vi "Get-Ctrl-Ref's & Label's.vi"(0 "VI Refnum":refnum<vi>, 7 "Show All Label List":bool, 11 "error in (no error)":errorcluster) -> (4 "Quick-GUI-Update out":refnum<class "Quick-GUI-Update.lvclass">, 8 "Label's List":string[][](array[string]), 15 "error out":errorcluster)   [LabVIEW 2020, in "Easy GUI Operation.lvlib" / "Quick-GUI-Update.lvclass"]
uses:
  Quick-GUI-Update.lvclass
  Quick-GUI-Update.lvclass/Quick-GUI-Update.ctl
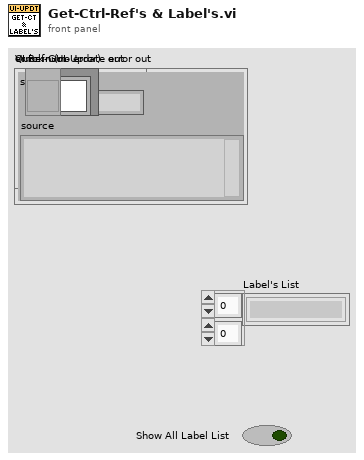
[diagram p1: front panel]
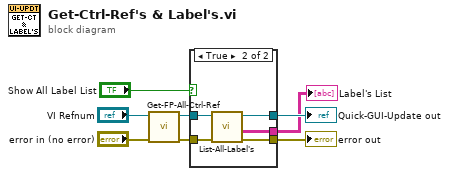
[diagram p0: block diagram]
diagram:
  n1 = call "Get-FP-All-Ctrl-Ref.vi"("error in (no error)"="error in (no error)", "VI Refnum"="VI Refnum") -> ("error out"=w3:errorcluster, "Quick-GUI-Update out"=w2:refnum<class "Quick-GUI-Update.lvclass">)  [unwired: 8 in]
  n2 = case shown="True" "Show All Label List" {
    tunnel: [w9 w15] -> w7
    tunnel: [w10 w14] -> w6
    tunnel: [_ w13] -> w4
    tunnel: w3 -> [w9 w12]
    tunnel: w2 -> [w10 w11]
    frame False {
    }
    frame True {
      n3 = call "List-All-Label's.vi"("error in (no error)"=w12, "Quick-GUI-Update in"=w11) -> ("error out"=w15:errorcluster, "Label's List"=w13:string[][], "Quick-GUI-Update out"=w14:refnum<class "Quick-GUI-Update.lvclass">)  [unwired: 7 in]
    }
  }
  "error out" <- w7
  "Quick-GUI-Update out" <- w6
  "Label's List" <- w4
